vi "Set JSON CFG.vi"(10 "<JSON> CFG":string, 11 "CFG JSON in":refnum<class "CFG JSON.lvclass">) -> (3 "CFG JSON out":refnum<class "CFG JSON.lvclass">)   [LabVIEW 2023, in "HAL.lvlib" / "CFG JSON.lvclass"]
uses:
  CFG JSON.lvclass
  CFG JSON.lvclass/CFG JSON.ctl
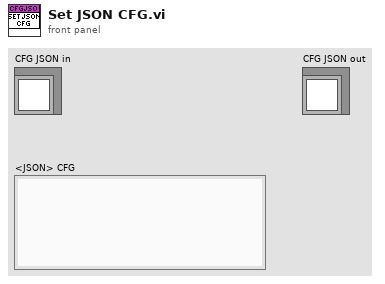
[diagram p1: front panel]
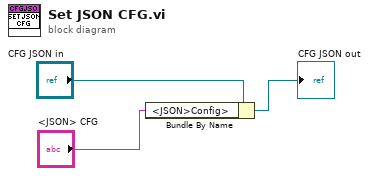
[diagram p0: block diagram]
diagram:
  n1 = Bundle By Name(cluster="CFG JSON in", "<JSON>Config>"="<JSON> CFG") -> (→"CFG JSON out":refnum<class "CFG JSON.lvclass">)
